vi "TextControlledInstrumControlChanged.vi"(0 "CtlRef":refnum<vi>, 1 "Control to Index":T1(c390), 2 "Command Array":string[][](array[string]), 3 "timeout in ms (1000ms)":i32=1000, 5 "OldVal":variant, 7 "NewVal":variant, 9 "IO Queue":refnum<queue>) -> ()   [LabVIEW 2020]
uses:
  TextControlledInstrumIOQueuePacket.ctl
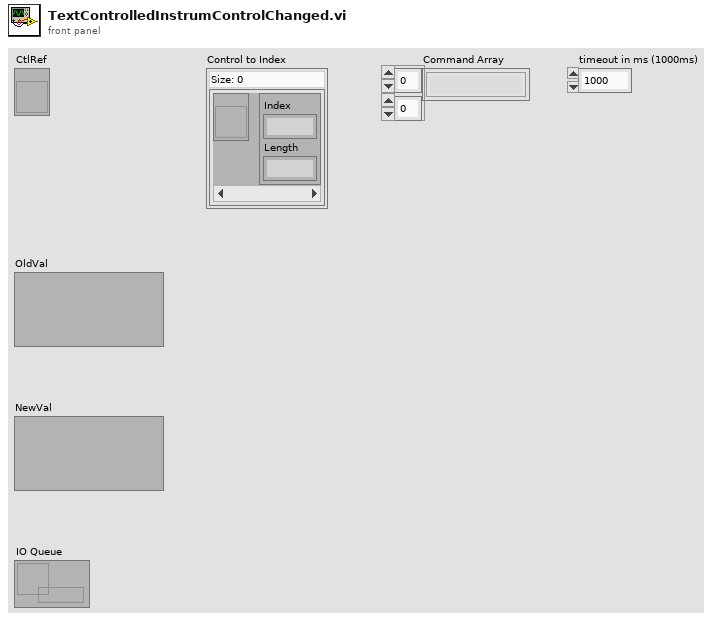
[diagram p1: front panel]
types:
  T1 = map{refnum<vi>, cluster{"Index":i32, "Length":i32}}
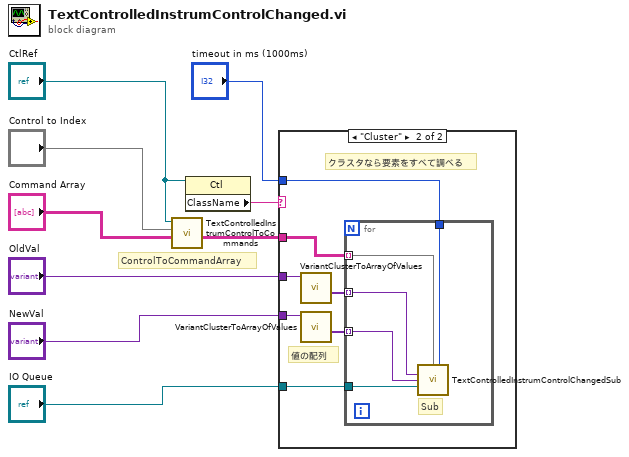
[diagram p0: block diagram]
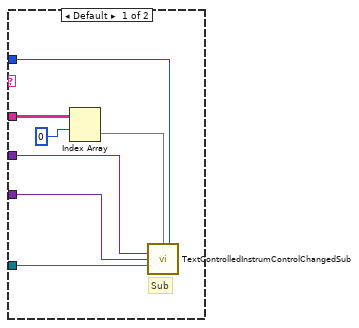
[diagram p2: hidden frame]
diagram:
  # "ControlToCommandArray"
  n1 = call "TextControlledInstrumControlToCommands.vi"("Command Array"="Command Array", "Control to Index"="Control to Index", "Control in"="CtlRef") -> ("Command Array out"=w5:string[][])  [unwired: 7 in, 1 out]
  n2 = property class="Ctl"(reference="CtlRef") -> ("ClassName"=w6:string)  [unwired: 1 in, 2 out]
  n3 = case shown="\"Cluster\"" w6 {
    tunnel: w5 -> [w16 w19]
    tunnel: "OldVal" -> [w10 w21]
    tunnel: "NewVal" -> [w11 w20]
    tunnel: "timeout in ms (1000ms)" -> [w14 w18]
    tunnel: "IO Queue" -> [w12 w17]
    frame Default {
      # "Sub"
      n4 = Index Array(array=w16, index (row)=0) -> (element=w13:string[])  [unwired: 1 in]
      n5 = call "TextControlledInstrumControlChangedSub.vi"("Command Array"=w13, "timeout in ms (1000ms)"=w14, "OldVal"=w10, "NewVal"=w11, "IO Queue"=w12) -> ()  [unwired: 11 in]
    }
    frame "Cluster" {
      # "クラスタなら要素をすべて調べる"
      # "値の配列"
      n6 = call "VariantClusterToArrayOfValues.vi"("Cluster Variant"=w21) -> ("Values"=w23:variant[])  [unwired: 8 in, 2 out]
      n7 = call "VariantClusterToArrayOfValues.vi"("Cluster Variant"=w20) -> ("Values"=w22:variant[])  [unwired: 8 in, 2 out]
      n8 = for {
        tunnel: w23 -> [w24] mode=indexing
        tunnel: w22 -> [w25] mode=indexing
        tunnel: w17 -> [w26]
        tunnel: w18 -> [w28]
        tunnel: w19 -> [w27] mode=indexing
        # "Sub"
        n9 = call "TextControlledInstrumControlChangedSub.vi"("Command Array"=w27, "timeout in ms (1000ms)"=w28, "OldVal"=w24, "NewVal"=w25, "IO Queue"=w26) -> ()  [unwired: 11 in]
      }
    }
  }
